vi "FTW-Benchmark-ProducerConsumer.vi"() -> ()   [LabVIEW 2013]
uses:
  source/actor/Message/Base/FTW-Message.lvclass
  source/actor/Producer/FTW-Producer.lvclass
  source/actor/Ether/FTW-Ether.lvclass
  source/actor/Consumer/FTW-Consumer.lvclass
panel:
  in  "Client Mode":enum32{"Parallel", "Serial"}(radio)=enum."Serial"
  in  "Number of Producers":i32=8
  out "Results":T1(array[cluster])
  in  "Server Addresses to Test":string[](array[string])=["tcp://127.0.0.1/*", "inproc://*"]
  in  "Messages to Send":i32=500
  in  "stop":bool
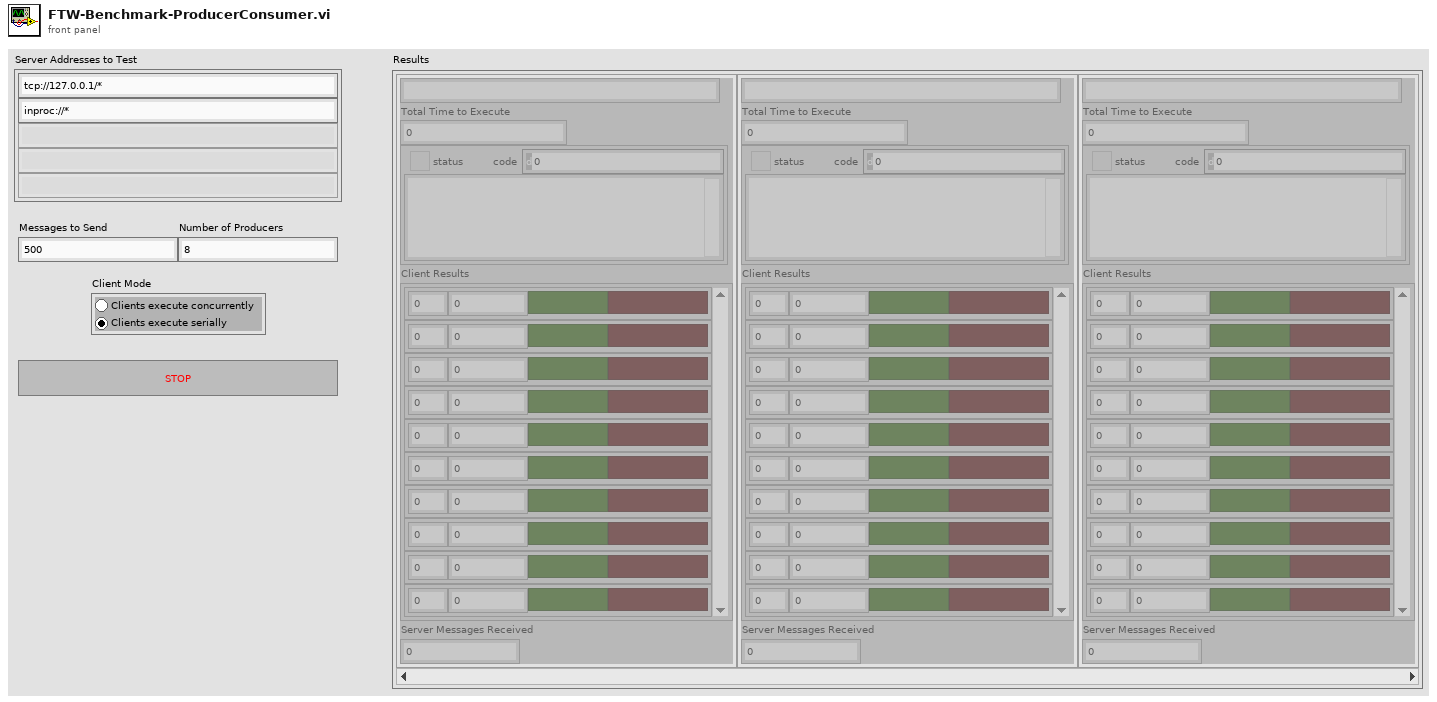
[diagram p1: front panel]
types:
  T1 = cluster{"Server Address":string, "Total Time to Execute":u32, "error":errorcluster, "Client Results":cluster{"Instance":i32, "Requests":i32, "All replies were as expected?":bool, "Timed out?":bool}[], "Server Messages Received":i32}[]
  T2 = cluster{"Actual Endpoint Address":string, "Elapsed Time":u32, "error out":errorcluster, cluster{i32, i32, bool, bool}[], i32}[]
  T3 = cluster{"Actual Address":string, "Elapsed Time":u32, "error IO":errorcluster, cluster{i32, i32, bool, bool}[], i32}
  T4 = cluster{"Actual Address":string, "Elapsed Time":u32, "error IO":errorcluster, cluster{i32, i32, bool, bool}[], i32}[]
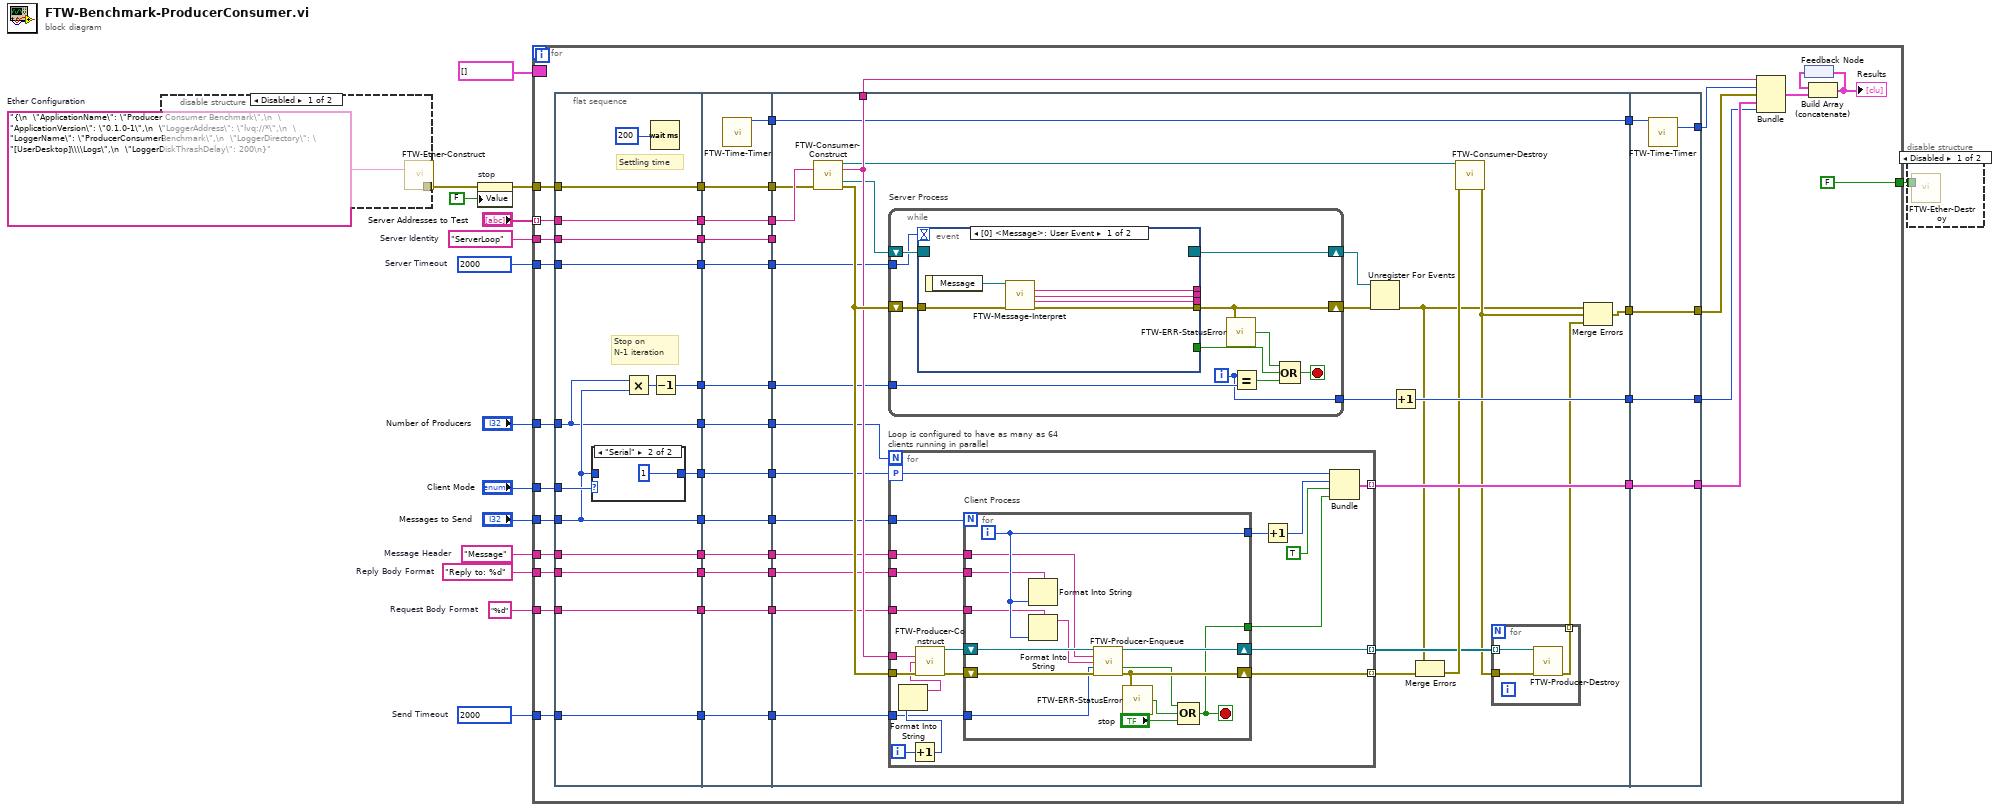
[diagram p0: block diagram]
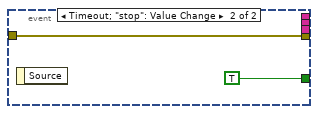
[diagram p5: hidden frame]
diagram:
  w1 = 2000  # Send Timeout
  w3 = "%d"  # Request Body Format
  w5 = "Message"  # Message Header
  w4 = "Reply to: %d"  # Reply Body Format
  w8 = 2000  # Server Timeout
  w12 = "ServerLoop"  # Server Identity
  n1 = disable-structure shown="Disabled" {
    disable-tunnel: [w17 _] -> w6
    frame Disabled {
      w16 = "{\n  \"ApplicationName\": \"Producer Consumer Benchmark\",\n  \"ApplicationVersion\": \"0.1.0-1\",\n  \"LoggerAddress\": \"lvq://*\",\n  \"LoggerName\": \"ProducerConsumerBenchmark\",\n  \"LoggerDirectory\": \"[UserDesktop]\\\\Logs\",\n  \"LoggerDiskThrashDelay\": 200\n}"  # Ether Configuration
      n2 = call "FTW-Ether-Construct.vi"("FTW Ether Configuration"=w16) -> ("error out"=w17:errorcluster)  [unwired: 14 in]
    }
    frame Enabled {
    }
  }
  n3 = property on="stop" class="Bool (strict)"(error in=w6, "Value"=FALSE ("stop")) -> (error out=w9:errorcluster)  [unwired: 1 in, 1 out]
  n4 = for {
    tunnel: "Server Addresses to Test" -> [w59] mode=indexing
    tunnel: "Number of Producers" -> [w54]
    tunnel: "Messages to Send" -> [w47]
    tunnel: w12 -> [w43]
    tunnel: "Client Mode" -> [w42]
    tunnel: w9 -> [w41]
    tunnel: w8 -> [w38]
    border: T2 [] -> [_]
    tunnel: w5 -> [w28]
    tunnel: w4 -> [w25]
    tunnel: w3 -> [w22]
    tunnel: [FALSE ("Force Destroy?")] -> w2
    tunnel: w1 -> [w18]
    n5 = flat-sequence {
      tunnel: [w81] -> w66
      tunnel: [w79] -> w60
      tunnel: [w68] -> w55
      tunnel: [w72] -> w48
      tunnel: [w78] -> w44
      tunnel: w41 -> [w81]
      tunnel: w42 -> [w76]
      tunnel: w43 -> [w78]
      tunnel: w47 -> [w72]
      tunnel: w54 -> [w68]
      tunnel: w59 -> [w79]
      tunnel: [w77] -> w39
      tunnel: w38 -> [w77]
      tunnel: [w75] -> w36
      tunnel: [w73] -> w34
      tunnel: [w71] -> w29
      tunnel: w28 -> [w71]
      tunnel: [w70] -> w26
      tunnel: w25 -> [w70]
      tunnel: [w69] -> w23
      tunnel: w22 -> [w69]
      tunnel: [w67] -> w19
      tunnel: w18 -> [w67]
      tunnel: [w96] -> w65
      tunnel: [w95] -> w64
      tunnel: w66 -> [w96]
      tunnel: [w94] -> w61
      tunnel: w60 -> [w94]
      tunnel: [w93] -> w56
      tunnel: w55 -> [w93]
      tunnel: [w92] -> w49
      tunnel: w48 -> [w92]
      tunnel: [w91] -> w45
      tunnel: w44 -> [w91]
      tunnel: [w90] -> w40
      tunnel: w39 -> [w90]
      tunnel: [w89] -> w37
      tunnel: w36 -> [w89]
      tunnel: [w88] -> w35
      tunnel: w34 -> [w88]
      tunnel: [w87] -> w30
      tunnel: w29 -> [w87]
      tunnel: [w86] -> w27
      tunnel: w26 -> [w86]
      tunnel: [w85] -> w24
      tunnel: w23 -> [w85]
      tunnel: [w84] -> w20
      tunnel: w19 -> [w84]
      tunnel: [w105] -> w63
      tunnel: [w122] -> w62
      tunnel: [w121] -> w52
      tunnel: [w120] -> w51
      tunnel: w35 -> [w116]
      tunnel: w37 -> [w108]
      tunnel: w65 -> [w106]
      tunnel: w64 -> [w122]
      tunnel: w61 -> [w107]
      tunnel: w56 -> [w113]
      tunnel: w49 -> [w115]
      tunnel: [w123] -> w46
      tunnel: w45 -> [_]
      tunnel: w40 -> [w112]
      tunnel: w30 -> [w104]
      tunnel: w27 -> [w103]
      tunnel: w24 -> [w102]
      tunnel: w20 -> [w101]
      tunnel: [w185] -> w58
      tunnel: w63 -> [w185]
      tunnel: w62 -> [w184]
      tunnel: [w183] -> w57
      tunnel: [w182] -> w53
      tunnel: w52 -> [w182]
      tunnel: [w181] -> w50
      tunnel: w51 -> [w181]
      frame #0 {
        # "Stop on\nN-1 iteration"
        # "Settling time"
        n6 = case shown="\"Serial\"" w76 {
          tunnel: w72 -> [w82 _]
          tunnel: [w82 1 ("Requests to Send")] -> w75
          frame "Parallel" {
          }
          frame "Serial" {
          }
        }
        n7 = Multiply(x=w68, y=w72) -> (x*y=w74:i32)
        n8 = Wait (ms)(milliseconds to wait=u32 200) -> ()  [unwired: 1 out]
        n9 = Decrement(x=w74) -> (x-1=w73:i32)
      }
      frame #1 {
        n10 = call "FTW-Time-Timer.vi"() -> ("Current Tick Count"=w95:u32)  [unwired: 13 in, 2 out]
      }
      frame #2 {
        n11 = call "FTW-Consumer-Construct.vi"("Address"=w107, "error in"=w106) -> ("FTW-Consumer Out"=w111:refnum<class "FTW-Consumer.lvclass">, "Actual Address"=w123:string, "Event Registration Refnum"=w117:refnum<event-registration>, "error out"=w124:errorcluster)  [unwired: 10 in]
        n12 = while "Server Process" {
          shift-right: [w171] -> w118
          shift-left: w117 -> [w172]
          shift-right: [w169] -> w119
          shift-left: w124 -> [w170]
          tunnel: w116 -> [w164]
          tunnel: [w163] -> w114
          tunnel: w112 -> [w162]
          i -> [w163]
          stop <- w165 stop-if-true
          n13 = event shown="[0] <Message>: User Event" {
            selector: w172 -> [_ _]
            dyn-events: [_ _] -> w171
            timeout: w162 -> [_ _]
            tunnel: [_ TRUE] -> w167
            tunnel: w170 -> [w178 w179]
            tunnel: [w177 w179] -> w169
            tunnel: [w175 _] -> _
            tunnel: [w174 _] -> _
            tunnel: [w173 _] -> _
            event User Event {
              n14 = event-data() -> ("Message"=w176:refnum<class "FTW-Message.lvclass">)  [unwired: 1 in]
              n15 = call-dynamic "FTW-Message-Interpret.vi"("FTW Message"=w176, "error in"=w178) -> ("Sender Identity"=w175:string, "Message Header"=w174:string, "Message Body"=w173:string, "error out"=w177:errorcluster)  [unwired: 9 in, 1 out]
            }
            event Timeout; "stop": Value Change {
              n16 = event-data() -> ()  [unwired: 1 in, 1 out]
            }
          }
          n17 = call "FTW-ERR-StatusError.vi"("error to check"=w169) -> ("Error?"=w168:bool)
          n18 = Equal?(x=w163, y=w164) -> (x = y?=w166:bool)
          n19 = Compound Arithmetic op=OR(w168, w167, w166) -> (w165:bool)
        }
        n20 = for "Loop is configured to have as many as 64 clients running in parallel" {
          N: w113 -> [_]
          tunnel: w124 -> [w137]
          tunnel: w115 -> [w147]
          workers-P: w108 -> [w143]
          tunnel: [w129] -> w110 mode=indexing
          tunnel: [w146] -> w121 mode=indexing
          tunnel: w123 -> [w135]
          tunnel: w103 -> [w141]
          tunnel: w104 -> [w140]
          tunnel: w102 -> [w139]
          tunnel: w101 -> [w130]
          tunnel: [w128] -> w100 mode=indexing
          i -> [w132]
          n21 = Increment(x=w132) -> (x+1=w131:i32)
          n22 = Format Into String(w131) -> (resulting string=w133:string)  [unwired: 3 in, 1 out]
          n23 = call "FTW-Producer-Construct.vi"("Server Address"=w135, "Identity"=w133, "error in"=w137) -> ("FTW-Producer Out"=w138:refnum<class "FTW-Producer.lvclass">, "error out"=w136:errorcluster)  [unwired: 11 in]
          n24 = for "Client Process" {
            N: w147 -> [_]
            shift-right: [w159] -> w128
            shift-left: w138 -> [w161]
            tunnel: [w152] -> w144
            tunnel: [w155] -> w145
            tunnel: w141 -> [w154]
            tunnel: w140 -> [w150]
            tunnel: w139 -> [w153]
            shift-right: [w158] -> w129
            shift-left: w136 -> [w160]
            tunnel: w130 -> [w149]
            i -> [w155]
            stop <- w152 stop-if-true
            n25 = Format Into String(format string=w154, w155) -> ()  [unwired: 2 in, 2 out]
            n26 = Format Into String(format string=w153, w155) -> (resulting string=w151:string)  [unwired: 2 in, 1 out]
            n27 = call "FTW-Producer-Enqueue.vi"("FTW-Producer In"=w161, "Header"=w150, "Body"=w151, "Timeout"=w149, "error in"=w160) -> ("FTW-Producer Out"=w159:refnum<class "FTW-Producer.lvclass">, "Timed out?"=w148:bool, "error out"=w158:errorcluster)  [unwired: 7 in, 1 out]
            n28 = call "FTW-ERR-StatusError.vi"("error to check"=w158) -> ("Error?"=w157:bool)
            n29 = Compound Arithmetic op=OR(w148, w157, "stop") -> (w152:bool)
          }
          n30 = Increment(x=w145) -> (x+1=w142:i32)
          n31 = Bundle(w143, w142, TRUE, w144) -> (w146:cluster{i32, i32, bool, bool})  [unwired: 1 in]
        }
        n32 = Unregister For Events(event registration refnum=w118, error in=w119) -> (error out=w97:errorcluster)
        n33 = Increment(x=w114) -> (x+1=w120:i32)
        n34 = Merge Errors(w97, w110) -> (w109:errorcluster)
        n35 = call "FTW-Consumer-Destroy.vi"("FTW-Consumer In"=w111, "error in"=w109) -> ("error out"=w99:errorcluster)  [unwired: 13 in]
        n36 = for {
          tunnel: w100 -> [w127] mode=indexing
          tunnel: w99 -> [w126]
          tunnel: [w125] -> w98 mode=indexing
          n37 = call "FTW-Producer-Destroy.vi"("FTW-Producer In"=w127, "error in"=w126) -> ("error out"=w125:errorcluster)  [unwired: 13 in]
        }
        n38 = Merge Errors(w97, w99, w98) -> (w105:errorcluster)
      }
      frame #3 {
        n39 = call "FTW-Time-Timer.vi"("Initial Tick Count"=w184) -> ("Elapsed Time"=w183:u32)  [unwired: 12 in, 2 out]
      }
    }
    n40 = Bundle("Actual Address"=w46, "Elapsed Time"=w57, "error IO"=w58, w53, w50) -> (w33:T3)  [unwired: 1 in]
    n41 = feedback #1() -> (w32:T2)
    n42 = Build Array (concatenate)(w32, w33) -> (w31:T4)
    "Results" <- w31
    n43 = feedback-in #1(w31) -> ()
  }
  n44 = disable-structure shown="Disabled" {
    disable-tunnel: w2 -> [w186 _]
    frame Disabled {
      n45 = call "FTW-Ether-Destroy.vi"("Force Destroy?"=w186) -> ()  [unwired: 14 in, 1 out]
    }
    frame Enabled {
    }
  }
